vi "Translator.File.MatchStrings.vi"   [LabVIEW 2016]
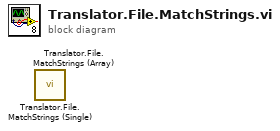
[diagram p0: block diagram]
diagram:
  n1 = call "Translator.File.MatchStrings (Single).vi"() -> ()  [unwired: 8 in, 4 out]
  n2 = call "Translator.File.MatchStrings (Array).vi"() -> ()  [unwired: 8 in, 4 out]
